vi "TCP - Engine.vi"() -> ()   [LabVIEW 2017]
uses:
  Controls/Read File.ctl
  Controls/RT- Queue States.ctl
  Controls/TCP - Test Settings.ctl
  Controls/TCP - Signals.ctl
  Controls/TCP - Signal Names.ctl
  Controls/TCP - Driver Control States.ctl
  SubVI - Global.vi
  Test cycle Execution/Control/Test Cycle Execution_States.ctl
panel:
  out "Waveform Chart":u32(graph)
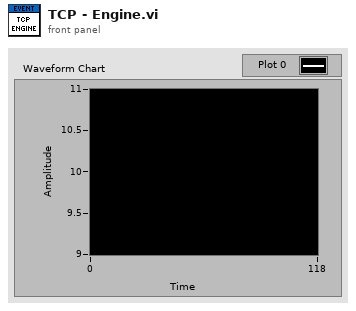
[diagram p1: front panel]
types:
  T1 = typedef "RT- Queue States.ctl" = enum16{"Initialize", "Enqueue", "Enqueue Priority", "Dequeue", "Flush", "Destroy"}
  T2 = typedef "Read File.ctl" = enum16{"Fetch XML", "Open", "Read", "Write", "Close"}
  T3 = typedef "TCP - Test Settings.ctl" = cluster{"Sequence File":string, "Iteration":i32}
  T4 = typedef "TCP - Signals.ctl" = cluster{"Signal":T5, "Value":bool, "Data":variant}
  T5 = typedef "TCP - Signal Names.ctl" = enum16{"Test Running", "Update Sensor Data", "Start Test", "Test Started", "Sequence Complete", "Seuence Aborted", "Abort Test", "Test Settings Updated", "Log Path", "Start Aux Logging", "Stop Aux Logging", "Reset Emergency", "Copy Log File", "Generate Alarm", "Download Files", "Send Test Details"}
  T6 = cluster{"Test details":cluster{"Furnace":string, "Material":string, "Angle":string, "ID":string, "Flowrate":string, "Test Name":string, "Tested By":string}, "Datalog Duration":dbl}
  T7 = typedef "Test Cycle Execution_States.ctl" = enum16{"Download Config Files", "Test Started", "Test Running", "Update Sensor Data", "Test Complete"}
  T8 = typedef "TCP - Driver Control States.ctl" = enum16{"Test Settings", "Send Test Details", "Boolean Commands", "Test Results"}
  T9 = cluster{"Furnace":string, "Material":string, "Angle":string, "ID":string, "Flowrate":string, "Test Name":string, "Tested By":string}
  T10 = typedef "TCP - Driver Control State.ctl" = enum16{"Test Settings", "Send Test Details", "Boolean Commands", "Test Results"}
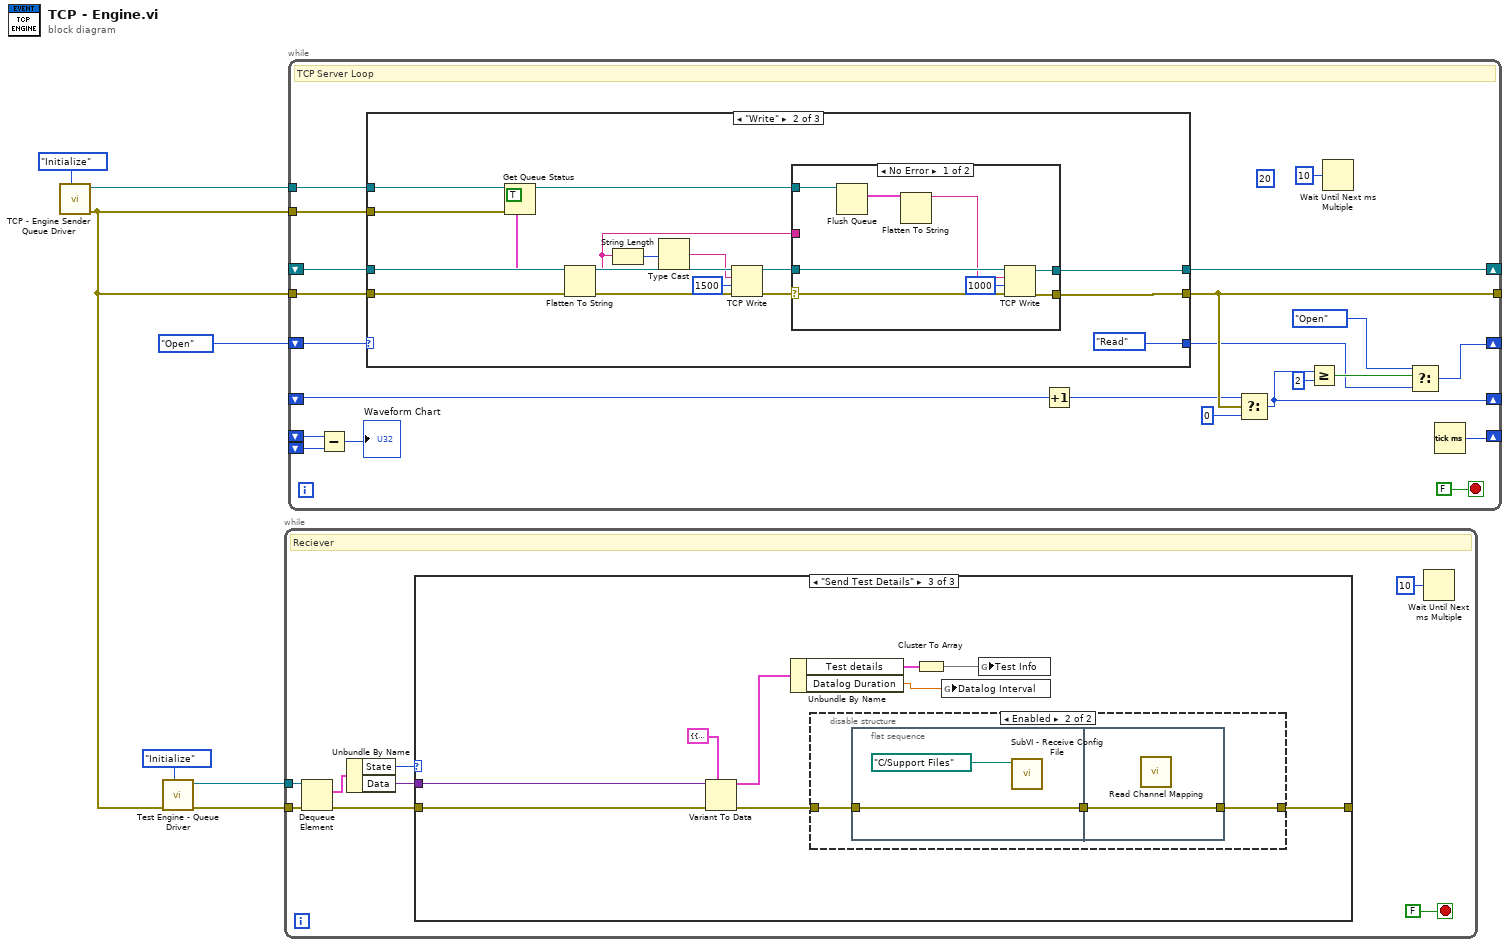
[diagram p0: block diagram]
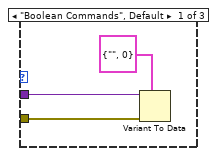
[diagram p2: hidden frame]
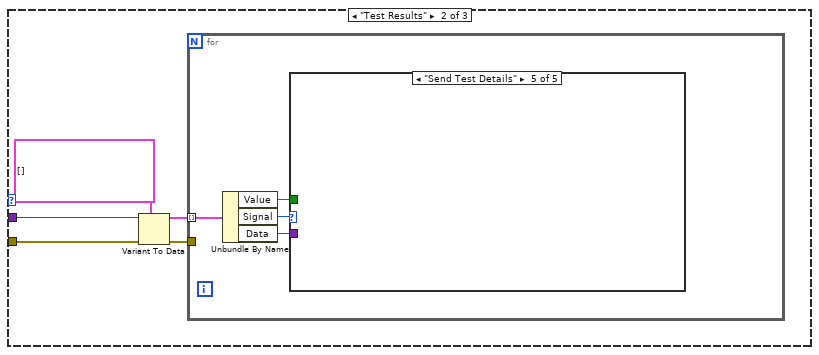
[diagram p3: hidden frame]
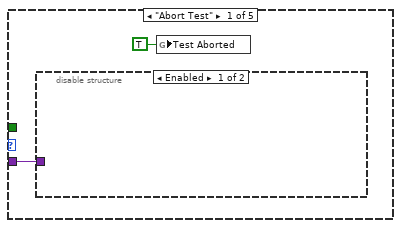
[diagram p4: hidden frame]
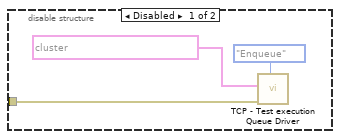
[diagram p9: hidden frame]
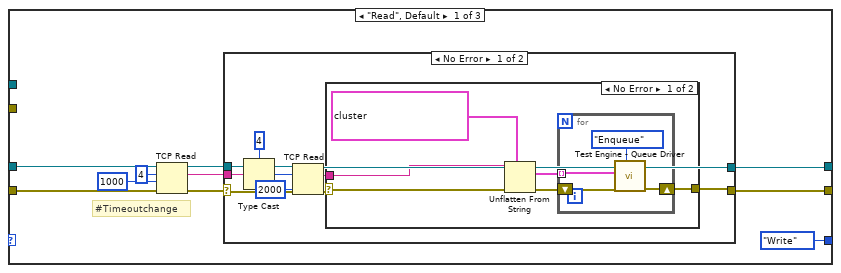
[diagram p10: hidden frame]
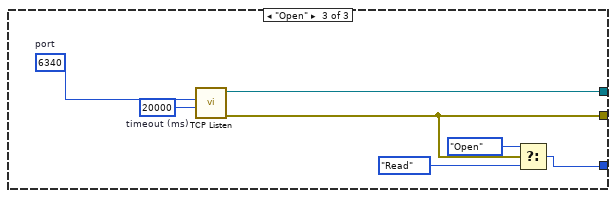
[diagram p14: hidden frame]
diagram:
  n1 = call "TCP - Engine Sender Queue Driver.vi"("Cases"=RT-_Queue_States."Initialize") -> ("error out"=w2:errorcluster, "queue out"=w1:refnum<queue>)  [unwired: 8 in, 1 out]
  n2 = call "Test Engine - Queue Driver.vi"("Cases"=RT-_Queue_States."Initialize", "error in (no error)"=w2) -> ("error out"=w4:errorcluster, "queue out"=w5:refnum<queue>)  [unwired: 7 in, 1 out]
  n3 = while {
    tunnel: w5 -> [w14]
    tunnel: w4 -> [w15]
    stop <- FALSE stop-if-true
    # "Reciever"
    n4 = Dequeue Element(queue=w14, error in (no error)=w15) -> (element=w12:cluster{"Data":variant, "State":T8}, error out=w13:errorcluster)  [unwired: 1 in, 2 out]
    n5 = Unbundle By Name(w12) -> ("State"=w10:T8, "Data"=w9:variant)
    n6 = case shown="\"Send Test Details\"" w10 {
      tunnel: w13 -> [w18 w22 w32]
      tunnel: w9 -> [w17 w23 w33]
      tunnel: [_ _ w30] -> _
      frame "Boolean Commands", Default {
        n7 = Variant To Data(error in=w18, type=T3 {"Sequence File"="", "Iteration"=0}, Variant=w17) -> ()  [unwired: 2 out]
      }
      frame "Test Results" {
        n8 = Variant To Data(error in=w22, type=T4[] [], Variant=w23) -> (data=w20:T4[], error out=w19:errorcluster)
        n9 = for {
          tunnel: w20 -> [w27] mode=indexing
          tunnel: w19 -> [_]
          n10 = Unbundle By Name(w27) -> ("Value"=w25:bool, "Signal"=w26:T5, "Data"=w24:variant)
          n11 = case shown="\"Send Test Details\"" w26 {
            tunnel: w25 -> [_ _ _ _ _]
            tunnel: w24 -> [w29 _ _ _ _]
            frame "Abort Test" {
              n12 = disable-structure shown="Enabled" {
                disable-tunnel: w29 -> [_ _]
                frame Enabled {
                }
                frame Disabled {
                }
              }
              n13 = global write "SubVI - Global.vi" "Test Aborted"(TRUE ("Test Aborted")) -> ()
            }
            frame "Stop Aux Logging" {
            }
            frame "Download Files", Default {
            }
            frame "Reset Emergency" {
            }
            frame "Send Test Details" {
            }
          }
        }
      }
      frame "Send Test Details" {
        n14 = Variant To Data(error in=w32, type=T6 {"Test details"={"Furnace"="Furnace A", "Material"="Aluminium", "Angle"="Multi Angle", "ID"="Trajectory 9", "Flowrate"="Flow", "Test Name"="Coke Burn", "Tested By"="Anirban"}, "Datalog Duration"=0.0}, Variant=w33) -> (data=w36:T6, error out=w31:errorcluster)
        n15 = Unbundle By Name(w36) -> ("Test details"=w35:T9, "Datalog Duration"=w34:dbl)
        n16 = disable-structure shown="Enabled" {
          disable-tunnel: w31 -> [w39 w43]
          disable-tunnel: [_ w42] -> w30
          frame Disabled {
            n17 = call "TCP - Test execution Queue Driver.vi"("Cases"=RT-_Queue_States."Enqueue", "error in (no error)"=w39, "Element In"=cluster{"Data":variant, "State":T7} {"Data"=variant, "State"=enum."Download Config Files"}) -> ()  [unwired: 6 in, 3 out]
          }
          frame Enabled {
            n18 = flat-sequence {
              tunnel: [w45] -> w44
              tunnel: w43 -> [w45]
              tunnel: w44 -> [w47]
              tunnel: [w47] -> w42
              frame #0 {
                n19 = call "SubVI - Receive Config File.vi"("file path (use dialog)"=path "C:/Support Files") -> ()  [unwired: 10 in, 1 out]
              }
              frame #1 {
                n20 = call "Read Channel Mapping.vi"() -> ()  [unwired: 12 in]
              }
            }
          }
        }
        n21 = Cluster To Array(cluster=w35) -> (array=w38:string[])
        n22 = global write "SubVI - Global.vi" "Datalog Interval"(w34) -> ()
        n23 = global write "SubVI - Global.vi" "Test Info"(w38) -> ()
      }
    }
    n24 = Wait Until Next ms Multiple(millisecond multiple=u32 10) -> ()  [unwired: 1 out]
  }
  n25 = while {
    shift-right: [w68] -> _
    shift-left: _ -> [w67]
    shift-right: [w57] -> _
    shift-left: Read_File."Open" ("R/W") -> [w69]
    shift-right: [w61] -> _
    shift-left: _ -> [w63]
    tunnel: w2 -> [w55]
    tunnel: w1 -> [w54]
    tunnel: w2 -> [w66]
    tunnel: [w65] -> _
    shift-right: [w51] -> _
    shift-left: _ -> [w50]
    shift-left: _ -> [w49]
    stop <- FALSE stop-if-true
    (unwired) u32 20 ("millisecond multiple")
    # "TCP Server Loop"
    n26 = Subtract(x=w50, y=w49) -> (x-y=→"Waveform Chart":u32)
    n27 = case shown="\"Write\"" w69 {
      tunnel: [w74 w116 w135] -> w68
      tunnel: [w73 w115 w134] -> w65
      tunnel: w67 -> [w79 w118 _]
      tunnel: w66 -> [w78 w108 _]
      tunnel: [Read_File."Write" ("R/W") Read_File."Read" ("R/W") w131] -> w53
      tunnel: w55 -> [_ w111 _]
      tunnel: w54 -> [_ w112 _]
      frame "Read", Default {
        # "#Timeoutchange"
        n28 = TCP Read(connection ID=w79, bytes to read=4, error in (no error)=w78, 9:1000 ("timeout ms (25000)")) -> (connection ID out=w77:refnum<k5>, data out=w72:string, error out=w70:errorcluster)  [unwired: 1 out]
        n29 = case shown="No Error" w70 {
          selector: w70 -> [w84 w101]
          tunnel: w77 -> [w89 w102]
          tunnel: [w88 w102] -> w74
          tunnel: [w83 w101] -> w73
          tunnel: w72 -> [w86 _]
          frame No Error {
            n30 = Type Cast(type=4 ("bytes to read"), x=w86) -> (*(type *) &x=w85:i32)
            n31 = TCP Read(connection ID=w89, bytes to read=w85, error in (no error)=w84, 9:2000 ("timeout ms (25000)")) -> (connection ID out=w88:refnum<k5>, data out=w82:string, error out=w81:errorcluster)  [unwired: 1 out]
            n32 = case shown="No Error" w81 {
              selector: w81 -> [w92 w100]
              tunnel: w82 -> [w93 _]
              tunnel: [w95 w100] -> w83
              frame No Error {
                n33 = Unflatten From String(type=cluster{"Data":variant, "State":T8}[] [{"Data"=variant, "State"=enum."Send Test Details"}], binary string=w93, error in (no error)=w92) -> (value=w90:cluster{"Data":variant, "State":T8}[], error out=w91:errorcluster)  [unwired: 2 in, 1 out]
                n34 = for {
                  tunnel: w90 -> [w96] mode=indexing
                  shift-right: [w98] -> w95
                  shift-left: w91 -> [w97]
                  n35 = call "Test Engine - Queue Driver.vi"("Cases"=RT-_Queue_States."Enqueue", "error in (no error)"=w97, "Element In"=w96) -> ("error out"=w98:errorcluster)  [unwired: 6 in, 2 out]
                }
              }
              frame Error {
              }
            }
          }
          frame Error {
          }
        }
      }
      frame "Write" {
        n36 = Get Queue Status(queue=w112, return elements? (F)=TRUE, error in (no error)=w111) -> (queue out=w103:refnum<queue>, elements=w109:cluster{"Data":variant, "State":T10}[])  [unwired: 6 out]
        n37 = Flatten To String(anything=w109, error in (no error)=w108) -> (data string=w104:string, error out=w107:errorcluster)  [unwired: 2 in, 1 out]
        n38 = String Length(string=w104) -> (length=w106:i32)
        n39 = Type Cast(x=w106) -> (*(type *) &x=w105:string)  [unwired: 1 out]
        n40 = TCP Write(connection ID=w118, data in=w105, error in (no error)=w107, 9:1500 ("timeout ms (25000)")) -> (connection ID out=w117:refnum<k5>, error out=w113:errorcluster)  [unwired: 1 out]
        n41 = case shown="No Error" w113 {
          selector: w113 -> [w124 w128]
          tunnel: w117 -> [w127 w129]
          tunnel: [w126 w129] -> w116
          tunnel: [w125 w128] -> w115
          tunnel: w104 -> [_ _]
          tunnel: w103 -> [w121 _]
          frame No Error {
            n42 = Flush Queue(queue=w121) -> (remaining elements=w122:cluster{"Data":variant, "State":T10}[])  [unwired: 1 in, 2 out]
            n43 = Flatten To String(anything=w122) -> (data string=w120:string)  [unwired: 3 in, 2 out]
            n44 = TCP Write(connection ID=w127, data in=w120, error in (no error)=w124, 9:1000 ("timeout ms (25000)")) -> (connection ID out=w126:refnum<k5>, error out=w125:errorcluster)  [unwired: 1 out]
          }
          frame Error {
          }
        }
      }
      frame "Open" {
        w130 = u16 6340  # port
        w136 = 20000  # timeout (ms)
        n45 = call <vilib>:"TCP Listen.vi"("timeout ms (wait forever: -1)"=w136, "port"=w130) -> ("error out"=w134:errorcluster, "connection ID"=w135:refnum<k5>)  [unwired: 5 in, 3 out]
        n46 = Select(t=Read_File."Open", s=w134, f=Read_File."Read" ("R/W")) -> (s? t:f=w131:T2)
      }
    }
    n47 = Increment(x=w63) -> (x+1=w62:i32)
    n48 = Select(t=w62, s=w65, f=0) -> (s? t:f=w61:i32)
    n49 = Greater Or Equal?(x=w61, y=2) -> (x >= y?=w58:bool)
    n50 = Wait Until Next ms Multiple(millisecond multiple=u32 10) -> ()  [unwired: 1 out]
    n51 = Select(t=Read_File."Open" ("f"), s=w58, f=w53) -> (s? t:f=w57:T2)
    n52 = Tick Count (ms)() -> (millisecond timer value=w51:u32)
  }
